vi "Initialize Data.vi"(8 "error in (no error)":errorcluster, 9 "data version":T1, 10 "data":string, 11 "Core Channel Configuration in":refnum<class "Core Channels Configuration.lvclass">) -> (0 "error out":errorcluster, 3 "Core Channel Configuration out":refnum<class "Core Channels Configuration.lvclass">)   [LabVIEW 2017, in "DSF Core.lvlib" / "Core Channels Configuration.lvclass"]
uses:
  Core Channels Configuration.lvclass
  Typedefs/DSF Version Info.ctl
  Core Channels Configuration.lvclass/Core Channels Configuration.ctl
  DSF Core.lvlib
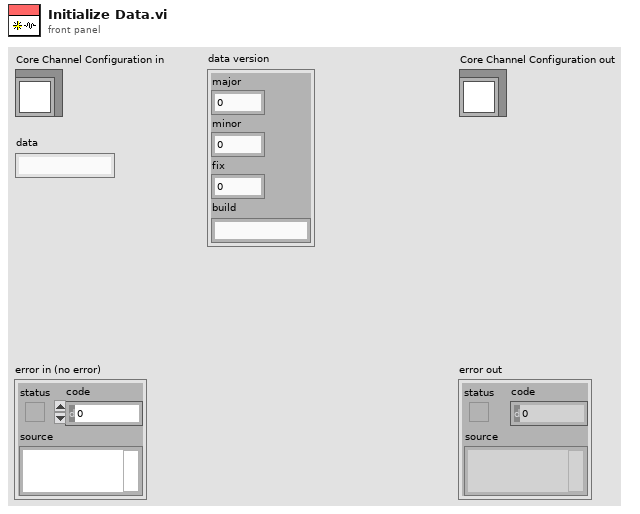
[diagram p1: front panel]
types:
  T1 = typedef "DSF Core.lvlib/DSF Version Info.ctl" = cluster{"major":i32, "minor":i32, "fix":i32, "build":string}
  T2 = cluster{"name":string, "units":string, "engine data type":enum8{"Bool", "SGL", "DBL", "I8", "I16", "I32", "I64", "U8", "U16", "U32", "U64"}, "string data type":enum8{"Bool", "SGL", "DBL", "I8", "I16", "I32", "I64", "U8", "U16", "U32", "U64"}, "string offset":u64}[]
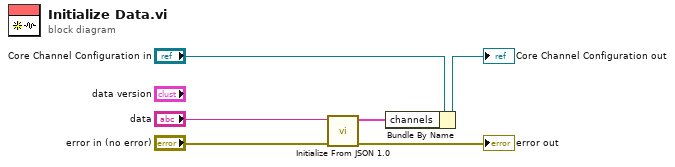
[diagram p0: block diagram]
diagram:
  n1 = call "Initialize From JSON 1.0.vi"("error in (no error)"="error in (no error)", "json"="data") -> ("error out"=→"error out":errorcluster, "channel configuration 1.0"=w3:T2)  [unwired: 8 in]
  n2 = Bundle By Name(cluster="Core Channel Configuration in", "channels"=w3) -> (→"Core Channel Configuration out":refnum<class "Core Channels Configuration.lvclass">)
